vi "Validate command.vi"(8 "error in (no error)":errorcluster, 10 "message":string, 11 "Motor in":refnum<class "Motor.lvclass">) -> (0 "error out":errorcluster, 1 "ack":bool, 3 "Motor out":refnum<class "Motor.lvclass">)   [LabVIEW 2018, in "Motor.lvclass"]
uses:
  Motor.lvclass
  Motor.lvclass/Motor.ctl
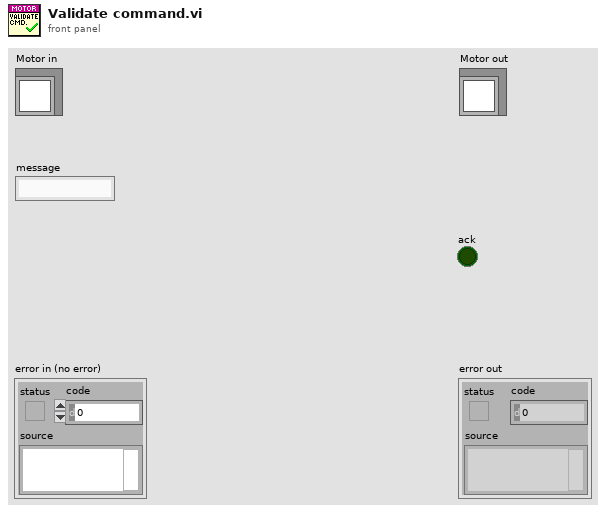
[diagram p1: front panel]
types:
  T1 = cluster{"action":string, "param":string, "pos_name":string, "pos_idx":i32, "ack":bool, "stop":bool, "offset":bool, "immediate":bool, "instructions":string[]}
  T2 = cluster{"mode":string, "condition":string, "position":string, "pos_name":string, "pos_id":string}
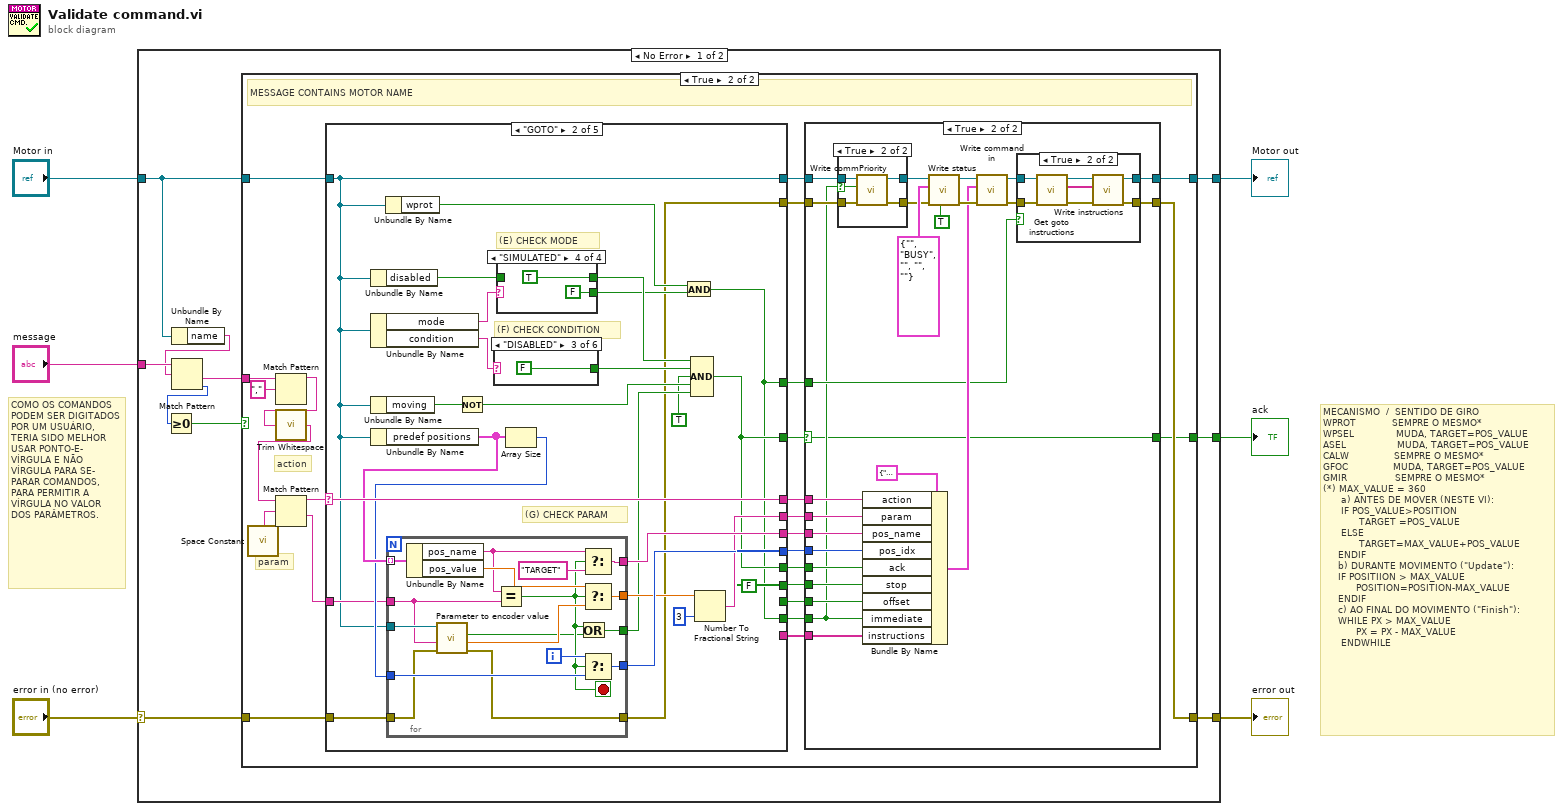
[diagram p0: block diagram]
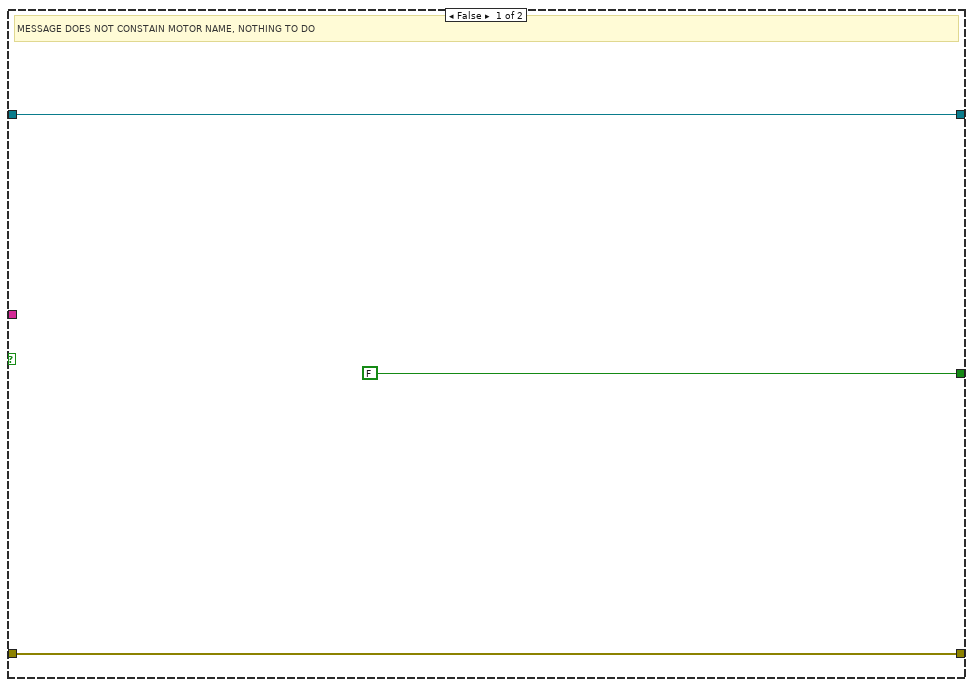
[diagram p2: hidden frame]
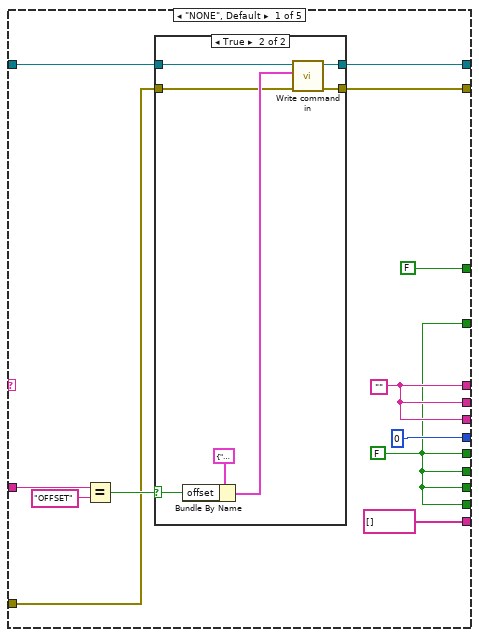
[diagram p6: hidden frame]
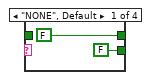
[diagram p8: hidden frame]
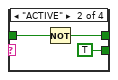
[diagram p9: hidden frame]
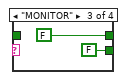
[diagram p10: hidden frame]
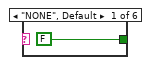
[diagram p11: hidden frame]
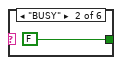
[diagram p12: hidden frame]
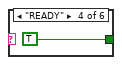
[diagram p13: hidden frame]
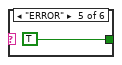
[diagram p14: hidden frame]
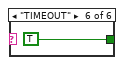
[diagram p15: hidden frame]
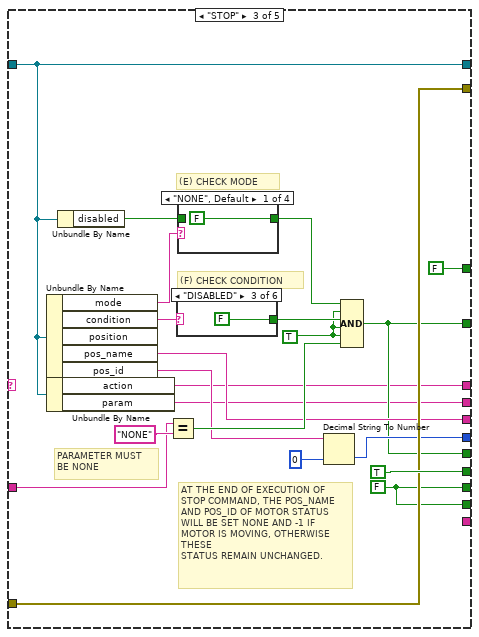
[diagram p16: hidden frame]
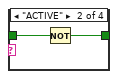
[diagram p17: hidden frame]
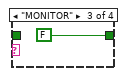
[diagram p18: hidden frame]
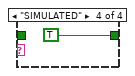
[diagram p19: hidden frame]
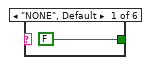
[diagram p20: hidden frame]
diagram:
  # "MECANISMO  /  SENTIDO DE GIRO\nWPROT            SEMPRE O MESMO*\nWPSEL              MUDA, TARGET=POS_VALUE\nASEL                 MUDA, TARGET=POS_VALUE\nCALW               SEMPRE O MESMO*\nGFOC               MUDA, TARGET=POS_VALUE\nGMIR                SEMPRE O MESMO*\n(*) MAX_VALUE = 360\n      a) ANTES DE MOVER (NESTE VI):\n      IF POS_VALUE>POSITION\n            TARGET =POS_VALUE\n      ELSE\n            TARGET=MAX_VALUE+POS_VALUE\n     ENDIF\n     b) DURANTE MOVIMENTO (\"Update\"):\n     IF POSITIION > MAX_VALUE\n           POSITION=POSITION-MAX_VALUE\n     ENDIF\n     c) AO FINAL DO MOVIMENTO (\"Finish\"):\n     WHILE PX > MAX_VALUE\n           PX = PX - MAX_VALUE\n      ENDWHILE"
  # "COMO OS COMANDOS PODEM SER DIGITADOS POR UM USUÁRIO, TERIA SIDO MELHOR \nUSAR PONTO-E-\nVÍRGULA E NÃO\nVÍRGULA PARA SE-\nPARAR COMANDOS,\nPARA PERMITIR A\nVÍRGULA NO VALOR\nDOS PARÂMETROS."
  n1 = case shown="No Error" "error in (no error)" {
    selector: "error in (no error)" -> [w9 w283]
    tunnel: [w8 w283] -> w5
    tunnel: [w10 w284] -> w2
    tunnel: "Motor in" -> [w12 w284]
    tunnel: "message" -> [w16 _]
    tunnel: [w7 _] -> w1
    frame No Error {
      n2 = Unbundle By Name(w12) -> ("name"=w15:string)
      n3 = Match Pattern(string=w16, regular expression=w15) -> (after substring=w13:string, offset past match=w14:i32)  [unwired: 1 in, 2 out]
      n4 = Greater Or Equal To 0?(x=w14) -> (x >= 0?=w11:bool)
      n5 = case shown="True" w11 {
        tunnel: w13 -> [_ w44]
        tunnel: w12 -> [w19 w38]
        tunnel: [w19 w31] -> w10
        tunnel: w9 -> [w18 w33]
        tunnel: [w18 w29] -> w8
        tunnel: [FALSE w20] -> w7
        frame False {
          # "MESSAGE DOES NOT CONSTAIN MOTOR NAME, NOTHING TO DO"
        }
        frame True {
          # "param"
          # "action"
          # "MESSAGE CONTAINS MOTOR NAME"
          n6 = call <vilib>:"Space Constant.vi"() -> ("String"=w41:string)
          n7 = Match Pattern(string=w44, regular expression=",") -> (before substring=w40:string)  [unwired: 1 in, 3 out]
          n8 = call <vilib>:"Trim Whitespace.vi"("string"=w40) -> ("trimmed string"=w42:string)  [unwired: 1 in]
          n9 = Match Pattern(string=w42, regular expression=w41) -> (before substring=w39:string, after substring=w27:string)  [unwired: 1 in, 2 out]
          n10 = case shown="\"GOTO\"" w39 {
            selector: w39 -> [_ w130 _ w216 w266]
            tunnel: w38 -> [w97 w112 w170 w201 w248]
            tunnel: [w98 w112 w170 w201 w248] -> w32
            tunnel: [w93 w116 w173 w205 w263] -> w26
            tunnel: [w93 w118 TRUE w203 w262] -> w37
            tunnel: [w100 w122 w168 w206 w246] -> w36
            tunnel: [w100 w129 w182 w207 ""] -> w35
            tunnel: [0 ("pos_idx") w131 w181 1 ("pos_idx") 0 ("pos_idx")] -> w34
            tunnel: w33 -> [w91 w119 w183 w202 w247]
            tunnel: [w92 w111 w183 w202 w247] -> w30
            tunnel: [w100 w130 w169 w216 w266] -> w28
            tunnel: w27 -> [w95 w120 w174 w206 w246]
            tunnel: [w93 w116 w173 w205 w263] -> w25
            tunnel: [w93 w118 w172 w203 w262] -> w24
            tunnel: [w93 w110 w172 w203 w244] -> w23
            tunnel: [string[] [] ("instructions") _ _ _ w240] -> w22
            tunnel: [FALSE w110 FALSE FALSE FALSE] -> w21
            frame "NONE", Default {
              w100 = ""
              w93 = FALSE
              n11 = Equal?(x=w95, y="OFFSET") -> (x = y?=w94:bool)
              n12 = case shown="True" w94 {
                selector: w94 -> [_ w107]
                tunnel: [w102 w109] -> w98
                tunnel: w97 -> [w102 w108]
                tunnel: [w101 w104] -> w92
                tunnel: w91 -> [w101 w103]
                frame False {
                }
                frame True {
                  n13 = Bundle By Name(cluster=T1 {"action"="", "param"="", "pos_name"="", "pos_idx"=0, "ack"=FALSE, "stop"=FALSE, "offset"=FALSE, "immediate"=FALSE, "instructions"=[]} ("command in"), "offset"=w107) -> (w105:T1)
                  n14 = call-dynamic "Write command in.vi"("error in (no error)"=w103, "command in"=w105, "Motor in"=w108) -> ("error out"=w104:errorcluster, "Motor out"=w109:refnum<class "Motor.lvclass">)  [unwired: 7 in]
                }
              }
            }
            frame "GOTO" {
              w118 = FALSE
              # "(E) CHECK MODE"
              # "(F) CHECK CONDITION"
              # "(G) CHECK PARAM"
              n15 = Unbundle By Name(w112) -> ("disabled"=w126:bool)
              n16 = Unbundle By Name(w112) -> ("mode"=w128:string, "condition"=w135:string)
              n17 = Unbundle By Name(w112) -> ("moving"=w133:bool)
              n18 = Unbundle By Name(w112) -> ("predef positions"=w125:cluster{"pos_name":string, "pos_value":dbl}[])
              n19 = Unbundle By Name(w112) -> ("wprot"=w114:bool)
              n20 = Not(x=w133) -> (.not. x?=w132:bool)
              n21 = case shown="\"DISABLED\"" w135 {
                tunnel: [FALSE FALSE FALSE TRUE TRUE TRUE] -> w134
                frame "NONE", Default {
                }
                frame "BUSY" {
                }
                frame "DISABLED" {
                }
                frame "READY" {
                }
                frame "ERROR" {
                }
                frame "TIMEOUT" {
                }
              }
              n22 = case shown="\"SIMULATED\"" w128 {
                tunnel: [FALSE w140 FALSE TRUE] -> w127
                tunnel: w126 -> [_ w139 _ _]
                tunnel: [FALSE TRUE FALSE FALSE] -> w115
                frame "NONE", Default {
                }
                frame "ACTIVE" {
                  n23 = Not(x=w139) -> (.not. x?=w140:bool)
                }
                frame "MONITOR" {
                }
                frame "SIMULATED" {
                }
              }
              n24 = Array Size(array=w125) -> (size(s)=w124:i32)
              n25 = for {
                tunnel: w125 -> [w161] mode=indexing
                tunnel: [w157] -> w123
                tunnel: [w158] -> w131
                tunnel: [w155] -> w129
                tunnel: w124 -> [w153]
                tunnel: w112 -> [w152]
                tunnel: [w148] -> w121
                tunnel: w120 -> [w147]
                tunnel: w119 -> [w146]
                tunnel: [w145] -> w111
                i -> [w159]
                stop <- w150 stop-if-true
                n26 = Unbundle By Name(w161) -> ("pos_name"=w156:string, "pos_value"=w160:dbl)
                n27 = call-dynamic "Parameter to encoder value.vi"("error in (no error)"=w146, "parameter"=w147, "Motor in"=w152) -> ("error out"=w145:errorcluster, "encoder value"=w151:dbl, "valid"=w149:bool)  [unwired: 5 in, 1 out]
                n28 = Equal?(x=w156, y=w147) -> (x = y?=w150:bool)
                n29 = Or(x=w150, y=w149) -> (x .or. y?=w148:bool)
                n30 = Select(t=w156, s=w150, f="TARGET") -> (s? t:f=w155:string)
                n31 = Select(t=w160, s=w150, f=w151) -> (s? t:f=w157:dbl)
                n32 = Select(t=w159, s=w150, f=w153) -> (s? t:f=w158:i32)
              }
              n33 = And(x=w114, y=w115) -> (x .and. y?=w110:bool)
              n34 = Compound Arithmetic op=AND(w127, w134, TRUE ("value"), w132, w121) -> (w116:bool)
              n35 = Number To Fractional String(number=w123, precision (6)=i16 3) -> (F-format string=w122:string)  [unwired: 2 in]
            }
            frame "STOP" {
              w172 = FALSE ("value")
              w177 = TRUE ("value")
              # "AT THE END OF EXECUTION OF STOP COMMAND, THE POS_NAME AND POS_ID OF MOTOR STATUS WILL BE SET NONE AND -1 IF MOTOR IS MOVING, OTHERWISE THESE\nSTATUS REMAIN UNCHANGED."
              # "PARAMETER MUST\nBE NONE"
              # "(E) CHECK MODE"
              # "(F) CHECK CONDITION"
              n36 = Unbundle By Name(w170) -> ("mode"=w178:string, "condition"=w188:string, "pos_name"=w182:string, "pos_id"=w179:string)  [unwired: 1 out]
              n37 = Unbundle By Name(w170) -> ("action"=w169:string, "param"=w168:string)
              n38 = Unbundle By Name(w170) -> ("disabled"=w175:bool)
              n39 = Equal?(x=w174, y="NONE") -> (x = y?=w185:bool)
              n40 = case shown="\"DISABLED\"" w188 {
                tunnel: [FALSE TRUE FALSE ("value") TRUE TRUE TRUE] -> w187
                frame "NONE", Default {
                }
                frame "BUSY" {
                }
                frame "DISABLED" {
                }
                frame "READY" {
                }
                frame "ERROR" {
                }
                frame "TIMEOUT" {
                }
              }
              n41 = case shown="\"NONE\", Default" w178 {
                tunnel: [FALSE w190 FALSE TRUE] -> w176
                tunnel: w175 -> [_ w191 _ _]
                frame "NONE", Default {
                }
                frame "ACTIVE" {
                  n42 = Not(x=w191) -> (.not. x?=w190:bool)
                }
                frame "MONITOR" {
                }
                frame "SIMULATED" {
                }
              }
              n43 = Decimal String To Number(string=w179, default (0L)=0 ("pos_idx")) -> (number=w181:i32)  [unwired: 1 in, 1 out]
              n44 = Compound Arithmetic op=AND(w176, w177, w187, w177, w177, w185) -> (w173:bool)
            }
            frame "INIT" {
              w211 = 1 ("index")
              w203 = FALSE
              # "PARAMETER MUST\nBE NONE"
              # "(E) CHECK MODE"
              # "(F) CHECK CONDITION"
              n45 = Unbundle By Name(w201) -> ("mode"=w225:string, "condition"=w224:string)
              n46 = Unbundle By Name(w201) -> ("moving"=w219:bool)
              n47 = Unbundle By Name(w201) -> ("predef positions"=w213:cluster{"pos_name":string, "pos_value":dbl}[])
              n48 = Unbundle By Name(w201) -> ("disabled"=w215:bool)
              n49 = Equal?(x=w206, y="NONE") -> (x = y?=w220:bool)
              n50 = Not(x=w219) -> (.not. x?=w218:bool)
              n51 = Array Size(array=w213) -> (size(s)=w212:i32)
              n52 = Index Array(array=w213, index=w211) -> (element=w214:cluster{"pos_name":string, "pos_value":dbl})
              n53 = case shown="\"ACTIVE\"" w225 {
                tunnel: [FALSE w230 w231 TRUE] -> w223
                tunnel: w215 -> [_ w229 _ _]
                tunnel: [FALSE TRUE w231 FALSE] -> _
                frame "NONE", Default {
                }
                frame "ACTIVE" {
                  n54 = Not(x=w229) -> (.not. x?=w230:bool)
                }
                frame "MONITOR" {
                  w231 = FALSE
                }
                frame "SIMULATED" {
                }
              }
              n55 = case shown="\"DISABLED\"" w224 {
                tunnel: [TRUE FALSE FALSE TRUE TRUE TRUE] -> w222
                frame "NONE", Default {
                }
                frame "BUSY" {
                }
                frame "DISABLED" {
                }
                frame "READY" {
                }
                frame "ERROR" {
                }
                frame "TIMEOUT" {
                }
              }
              n56 = Equal?(x=w212, y=w211) -> (x = y?=w208:bool)
              n57 = Unbundle By Name(w214) -> ("pos_name"=w210:string)
              n58 = Select(t="TARGET", s=w208, f=w210) -> (s? t:f=w207:string)
              n59 = Compound Arithmetic op=AND(w223, w222, TRUE ("value"), w218, w220) -> (w205:bool)
            }
            frame "CYCLIC" {
              w249 = u32 65535
              w262 = FALSE
              # "BITS 0-15 ENABLE WP1-16"
              # "(E) CHECK MODE"
              # "(F) CHECK CONDITION"
              n60 = Unbundle By Name(w248) -> ("mode"=w271:string, "condition"=w270:string)
              n61 = Unbundle By Name(w248) -> ("moving"=w269:bool)
              n62 = Unbundle By Name(w248) -> ("wprot"=w259:bool)
              n63 = Unbundle By Name(w248) -> ("disabled"=w264:bool)
              n64 = Decimal String To Number(string=w246, default (0L)=w249) -> (number=w258:u32)  [unwired: 1 in, 1 out]
              n65 = Not(x=w269) -> (.not. x?=w268:bool)
              n66 = Equal?(x=w246, y="SINGLE" ("x")) -> (x = y?=w254:bool)
              n67 = Equal?(x=w246, y="SEVERAL") -> (x = y?=w251:bool)
              n68 = Equal?(x=w246, y="START") -> (x = y?=w244:bool)
              n69 = And(x=w249, y=w258) -> (x .and. y?=w257:u32)
              n70 = Greater Than 0?(x=w257) -> (x > 0?=w255:bool)
              n71 = case shown="\"ACTIVE\"" w271 {
                tunnel: [FALSE w274 FALSE FALSE] -> w260
                tunnel: w264 -> [_ w273 _ _]
                frame "NONE", Default {
                }
                frame "ACTIVE" {
                  n72 = Not(x=w273) -> (.not. x?=w274:bool)
                }
                frame "MONITOR" {
                }
                frame "SIMULATED" {
                }
              }
              n73 = case shown="\"DISABLED\"" w270 {
                tunnel: [FALSE FALSE FALSE TRUE TRUE TRUE] -> w261
                frame "NONE", Default {
                }
                frame "BUSY" {
                }
                frame "DISABLED" {
                }
                frame "READY" {
                }
                frame "ERROR" {
                }
                frame "TIMEOUT" {
                }
              }
              n74 = Compound Arithmetic op=OR(w255, w254, w251, w244) -> (w253:bool)
              n75 = Build Array("SR1=1" ("string")) -> (w242:string[])
              n76 = Select(t=w242, s=w244, f=string[] [] ("instructions")) -> (s? t:f=w240:string[])
              n77 = Compound Arithmetic op=AND(w259, w260, w261, w268, w253) -> (w263:bool)
            }
          }
          n78 = case shown="True" w25 {
            selector: w25 -> [w45 w48]
            tunnel: w37 -> [_ w72]
            tunnel: w36 -> [_ w70]
            tunnel: w35 -> [_ w68]
            tunnel: w34 -> [_ w71]
            tunnel: w32 -> [w47 w53]
            tunnel: [w47 w56] -> w31
            tunnel: w30 -> [w46 w52]
            tunnel: [w46 w55] -> w29
            tunnel: w28 -> [_ w69]
            tunnel: w26 -> [_ w64]
            tunnel: w24 -> [_ w63]
            tunnel: w23 -> [_ w49]
            tunnel: w22 -> [_ w59]
            tunnel: w21 -> [_ w54]
            tunnel: [w45 w48] -> w20
            frame False {
            }
            frame True {
              n79 = case shown="True" w49 {
                selector: w49 -> [_ w75]
                tunnel: w53 -> [w74 w79]
                tunnel: w52 -> [w73 w76]
                tunnel: [w74 w78] -> w51
                tunnel: [w73 w77] -> w50
                frame False {
                }
                frame True {
                  n80 = call-dynamic "Write commPriority.vi"("error in (no error)"=w76, "commPriority"=w75, "Motor in"=w79) -> ("error out"=w77:errorcluster, "Motor out"=w78:refnum<class "Motor.lvclass">)  [unwired: 7 in]
                }
              }
              n81 = Bundle By Name(cluster=T1 {"action"="", "param"="", "pos_name"="", "pos_idx"=0, "ack"=FALSE, "stop"=FALSE, "offset"=FALSE, "immediate"=FALSE, "instructions"=[]} ("command in"), "action"=w69, "param"=w70, "pos_name"=w68, "pos_idx"=w71, "ack"=w64, "stop"=w72, "offset"=w63, "immediate"=w49, "instructions"=w59) -> (w60:T1)
              n82 = call-dynamic "Write status.vi"("hold if empty"=TRUE, "error in (no error)"=w50, "status"=T2 {"mode"="", "condition"="BUSY", "position"="", "pos_name"="", "pos_id"=""}, "Motor in"=w51) -> ("error out"=w66:errorcluster, "Motor out"=w67:refnum<class "Motor.lvclass">)  [unwired: 6 in]
              n83 = call-dynamic "Write command in.vi"("error in (no error)"=w66, "command in"=w60, "Motor in"=w67) -> ("error out"=w57:errorcluster, "Motor out"=w58:refnum<class "Motor.lvclass">)  [unwired: 7 in]
              n84 = case shown="True" w54 {
                tunnel: w58 -> [w81 w88]
                tunnel: w57 -> [w80 w87]
                tunnel: [w81 w83] -> w56
                tunnel: [w80 w85] -> w55
                frame False {
                }
                frame True {
                  n85 = call-dynamic "Get goto instructions.vi"("error in (no error)"=w87, "Motor in"=w88) -> ("error out"=w86:errorcluster, "goto instructions"=w82:string[], "Motor out"=w84:refnum<class "Motor.lvclass">)  [unwired: 6 in, 1 out]
                  n86 = call-dynamic "Write instructions.vi"("error in (no error)"=w86, "instructions"=w82, "Motor in"=w84) -> ("error out"=w85:errorcluster, "Motor out"=w83:refnum<class "Motor.lvclass">)  [unwired: 7 in]
                }
              }
            }
          }
        }
      }
    }
    frame Error {
    }
  }
  "error out" <- w5
  "Motor out" <- w2
  "ack" <- w1
